vi "Flow Module (Main).vi"(7 "Name of Parent Panel":string="Main.vi", 9 "New Center Coords":T2={"Horizontal"=470, "Vertical"=200}, 10 "Config":variant, 11 "Main UI Message Queue":refnum<queue>) -> ()   [LabVIEW 2018, in "Flow Module.lvlib"]
doc: "This Continuous Measurement sample project is based on the Queued Message Handler template.\n\nThe Event Handling Loop generates messages based on user interface actions.\n\nThe Message Handling Loop processes messages generated by the Event Handling Loop, or by other messages. There are also Acquisition and Logging message handling loop subVIs, and a chart updating loop."
uses:
  Flow Module.lvlib
  support/Message Queue/Message Cluster.ctl
  <vilib>/Utility/miscctls.llb/LVPoint32TypeDef.ctl
  controls/UI State.ctl
  Feed Module/Controls/Flow Module State Cluster.ctl
  Feed Module/Controls/Flow Module Config Cluster.ctl
  Feed Module/Controls/Flow Module Settings Cluster.ctl
  Bronkhorst M13 Flow Meter/Settings Cluster.ctl
  Bronkhorst M14 Flow Meter/Settings Cluster.ctl
  Feed Module/Controls/Flow Module Display.ctl
  support/Message Queue/Enqueue Message (Single).vi
  support/User Event - Stop/User Event - Stop.lvlib
  support/Message Queue/Message Queue.lvlib
  support/Support Library.lvlib
  Measure Instrument/Flow Module Engine.lvlib
  support/Command Log VIs/Command Logging.lvlib
  Bronkhorst M14 Flow Meter/Bronkhorst M14 Flow Meter.lvlib
  Bronkhorst M13 Flow Meter/Bronkhorst M13 Flow Meter.lvlib
  Report Generation/Report Generation.lvlib
panel:
  in  "Settings Button":bool
  out "User Name":string
  out "Display Cluster":T1 {"Total g" format="%4.2f"; "C" format="%5.2f"; "kg/m^3" format="%6.1f"; "g/min" format="%4.2f"}
  out "Original Width":u32
  out "Original Height":u32
  out "H/W":dbl
  out "ScanCode":i16
  out "Log File path":path
  out "Status":string
  in  "Exit":bool
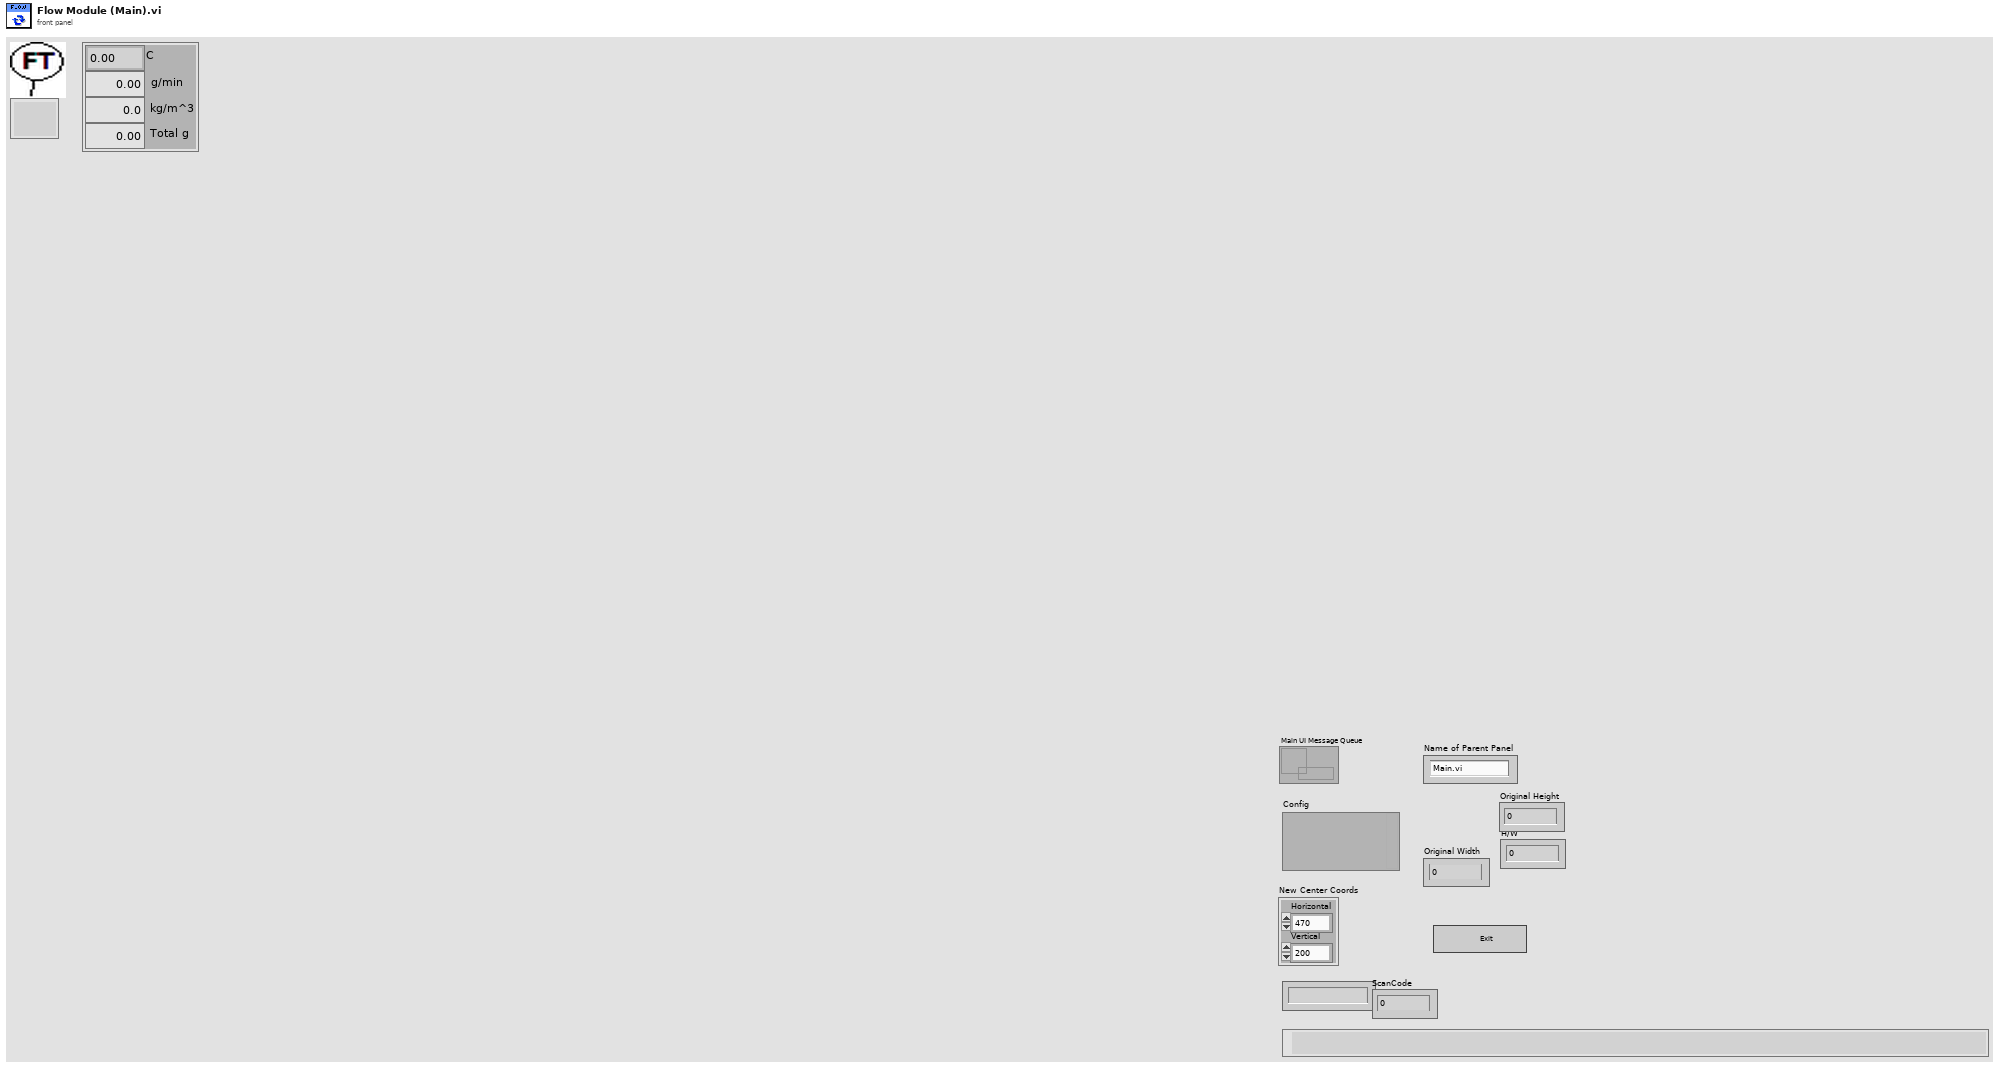
[diagram p1: front panel]
types:
  T1 = cluster{"C":dbl, "g/min":dbl, "kg/m^3":dbl, "Total g":dbl}
  T2 = typedef "LVPoint32TypeDef.ctl" = cluster{"Horizontal":i32, "Vertical":i32}
  T3 = enum32{"Invalid", "Default", "Floating", "Floating/Auto-Hide", "Modal"}
  T4 = typedef "Flow Module.lvlib/Flow Module Config Cluster.ctl" = cluster{"GUID":string, "Drop Coords":T2, "Process Name":string, "User name":string, "Queue Name":string, "Settings":T5, "Load Count":i32}
  T5 = typedef "Flow Module.lvlib/Flow Module Settings Cluster.ctl" = cluster{"Cycle Period":dbl, "Flow Meter Type":string, "Bronkhorst M13 Settings":T6, "Bronkhorst M14 Settings":T7, "Reset Totalizer":bool}
  T6 = typedef "Bronkhorst M13 Flow Meter.lvlib/Settings Cluster.ctl" = cluster{"VISA resource name":refnum<visa-resource-name>, "Simulated?":bool, "Smoothing Steps":i32}
  T7 = typedef "Bronkhorst M14 Flow Meter.lvlib/Settings Cluster.ctl" = cluster{"VISA resource name":refnum<visa-resource-name>, "Simulated?":bool, "Smoothing Steps":i32}
  T8 = typedef "UI State.ctl" = enum16{"Idle", "Acquiring and Logging", "Waiting for Exit", "Waiting for Exit (Acq Stopped)", "Waiting for Exit (Log Stopped)", "Waiting for Stop", "Waiting for Stop (Acq Stopped)", "Waiting for Stop (Log Stopped)"}
  T9 = typedef "Flow Module.lvlib/Flow Module State Cluster.ctl" = cluster{"Flow Module Config":T4}
  T10 = typedef "LVPointTypeDef.ctl" = cluster{"Horizontal":i16, "Vertical":i16}
  T11 = typedef "Flow Module.lvlib/Flow Message Queues.ctl" = cluster{"Flow UI":refnum<queue>, "Flow Engine":refnum<queue>, "Flow Display":refnum<queue>}
  T12 = typedef "Flow Module.lvlib/Flow Module Display.ctl" = cluster{"Flow Value":dbl, "Cycle Period":dbl, "Density":dbl, "Temp":dbl, "Totalized":dbl}
  T13 = typedef "LVRectTypeDef.ctl" = cluster{"Left":i16, "Top":i16, "Right":i16, "Bottom":i16}
  T14 = cluster{"Shift":bool, "Ctrl":bool, "Alt":bool, "Cmd":bool, "Opt":bool}
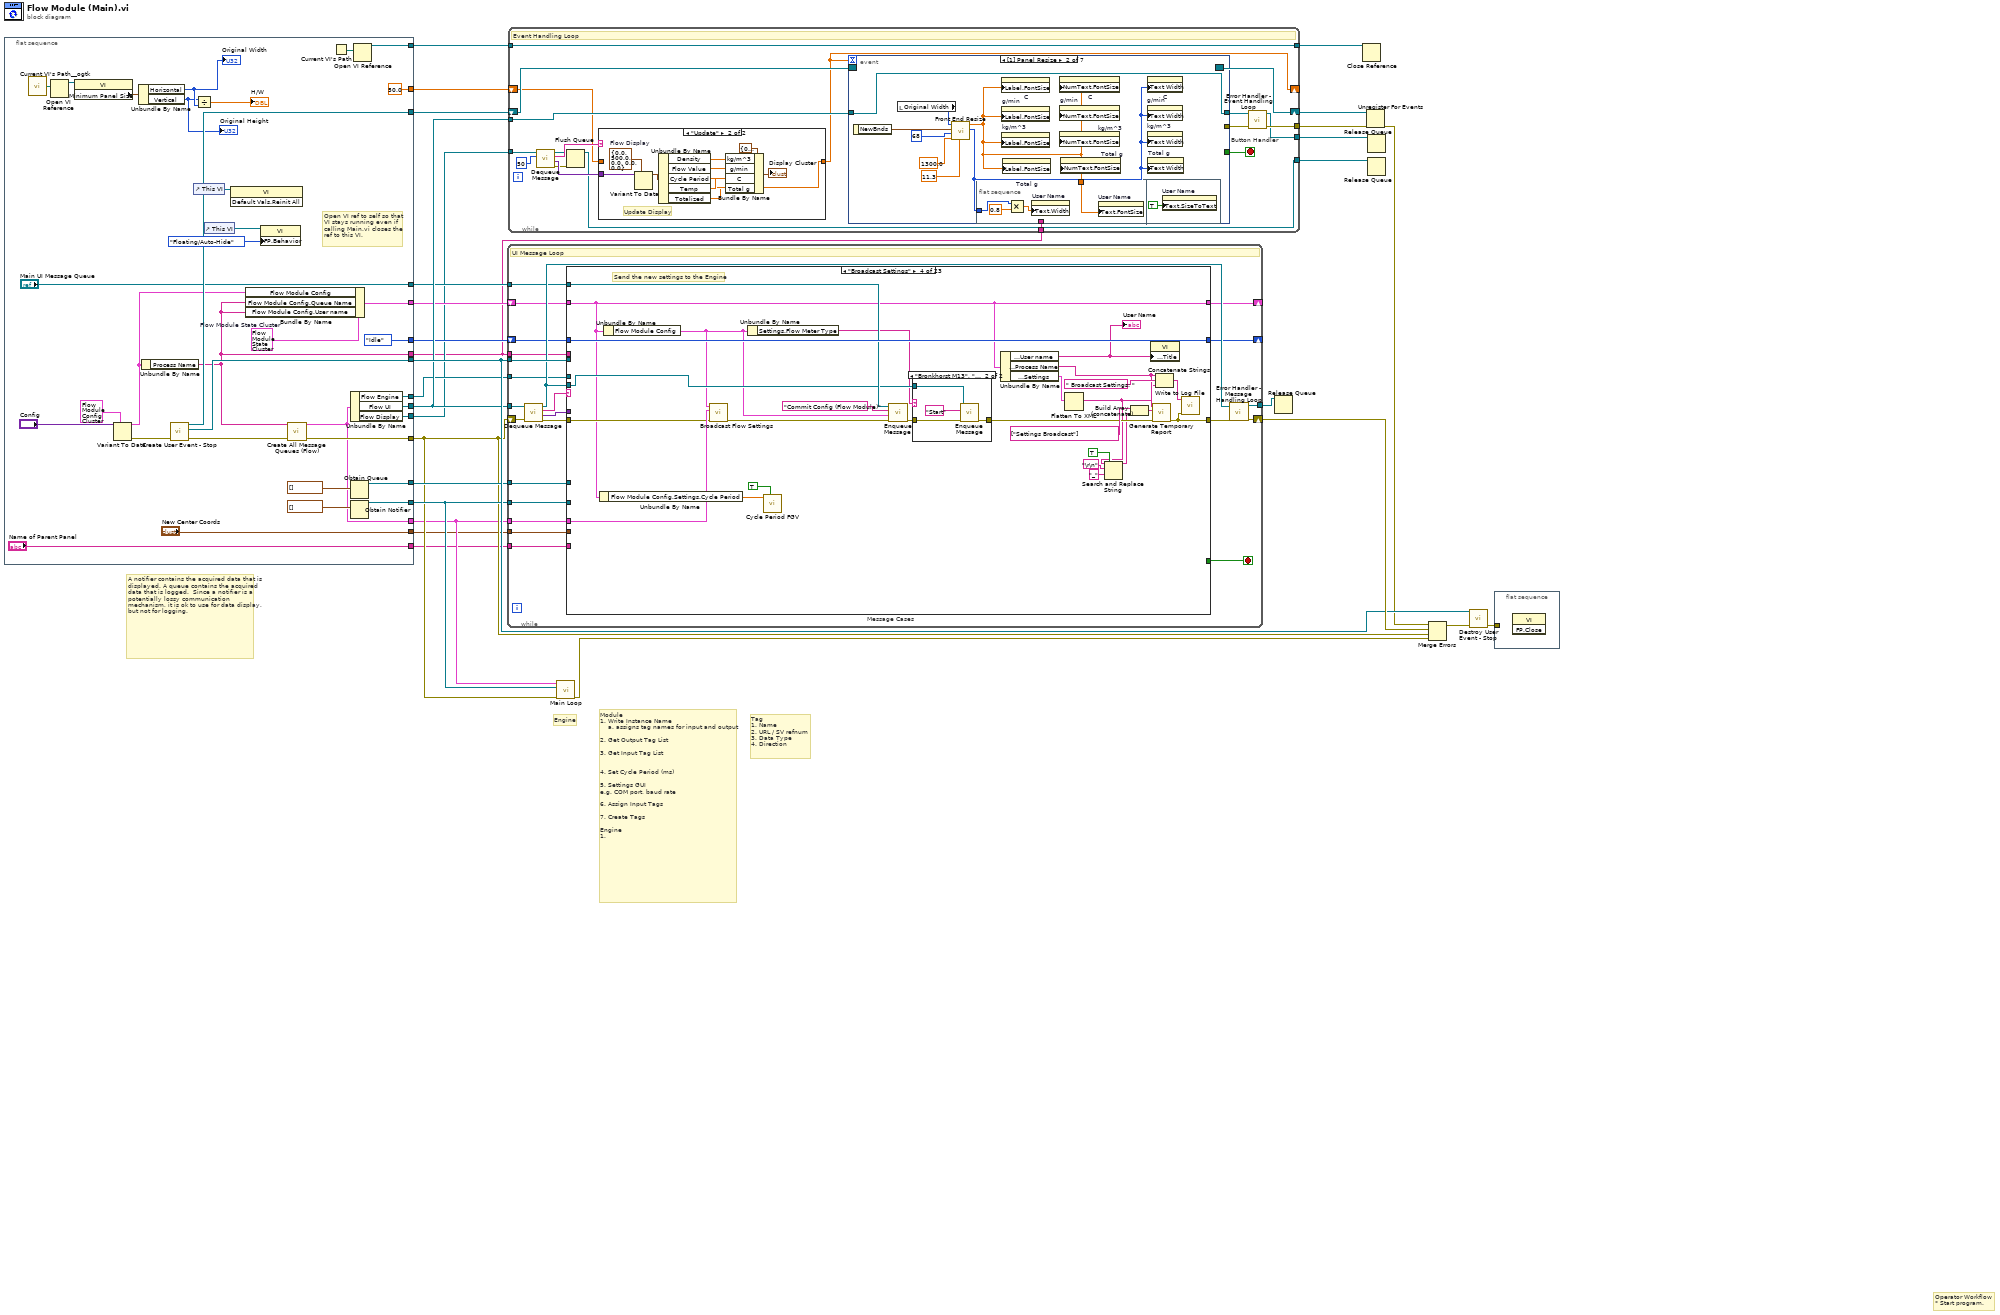
[diagram p0: block diagram]
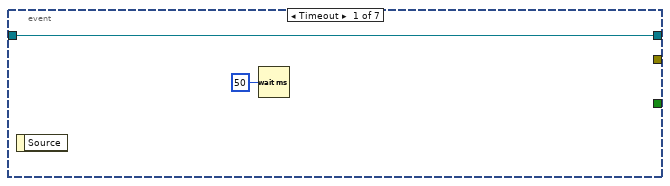
[diagram p3: hidden frame]
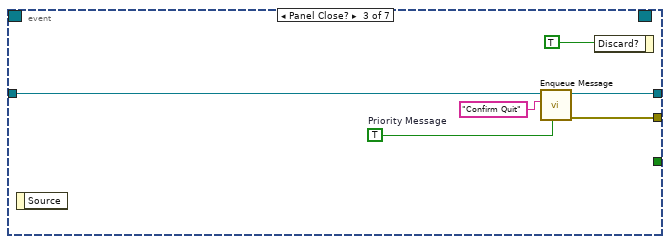
[diagram p4: hidden frame]
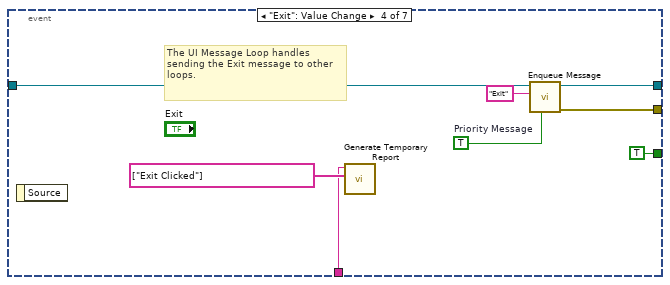
[diagram p5: hidden frame]
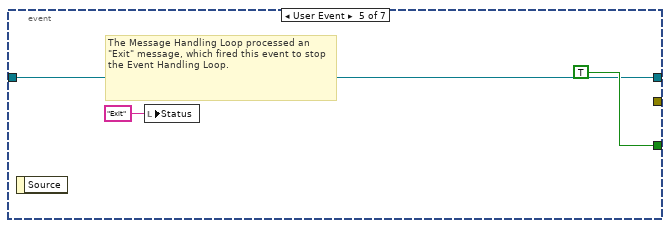
[diagram p6: hidden frame]
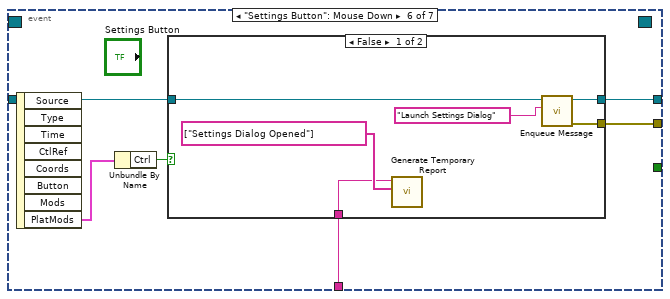
[diagram p7: hidden frame]
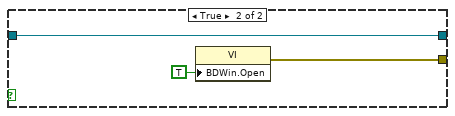
[diagram p8: hidden frame]
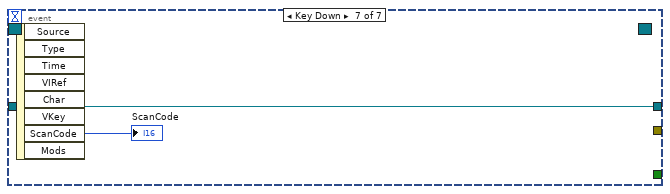
[diagram p9: hidden frame]
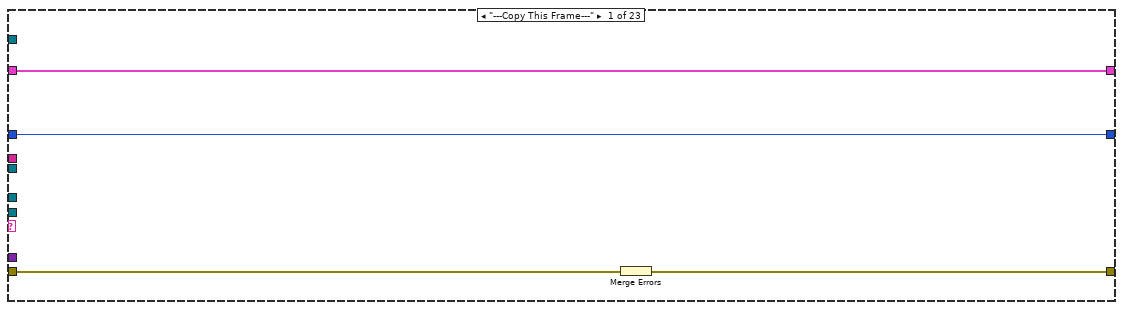
[diagram p10: hidden frame]
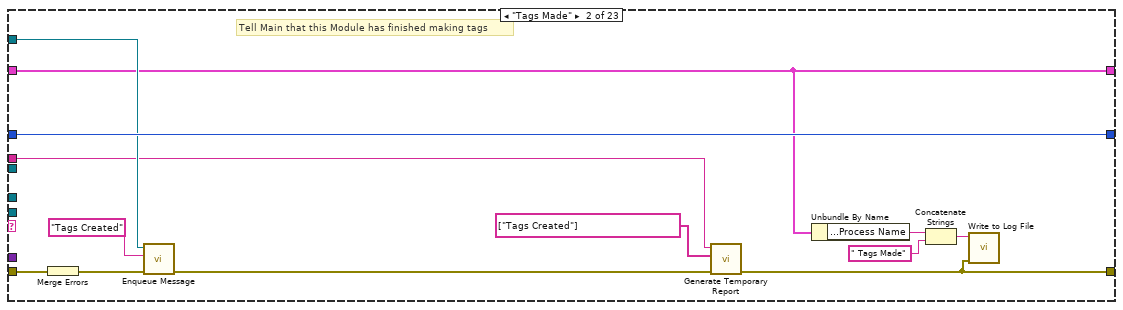
[diagram p11: hidden frame]
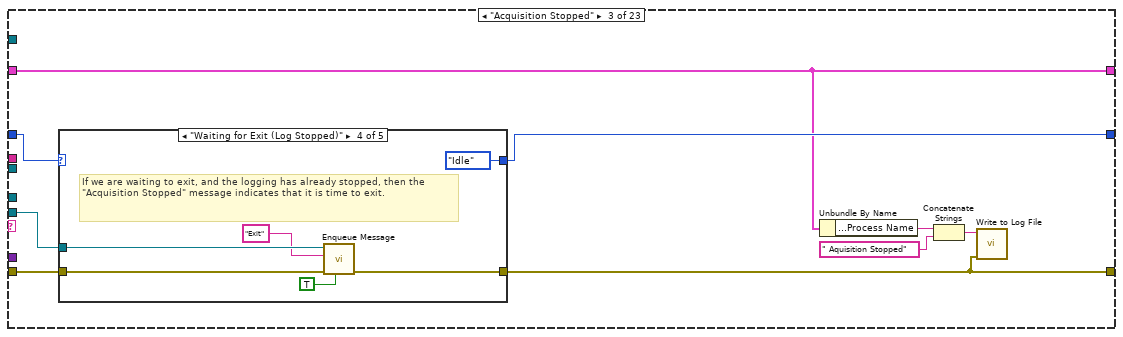
[diagram p12: hidden frame]
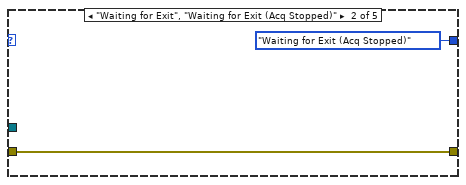
[diagram p14: hidden frame]
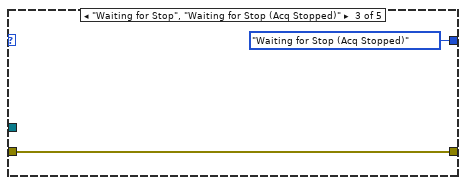
[diagram p15: hidden frame]
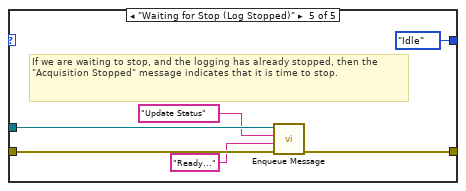
[diagram p16: hidden frame]
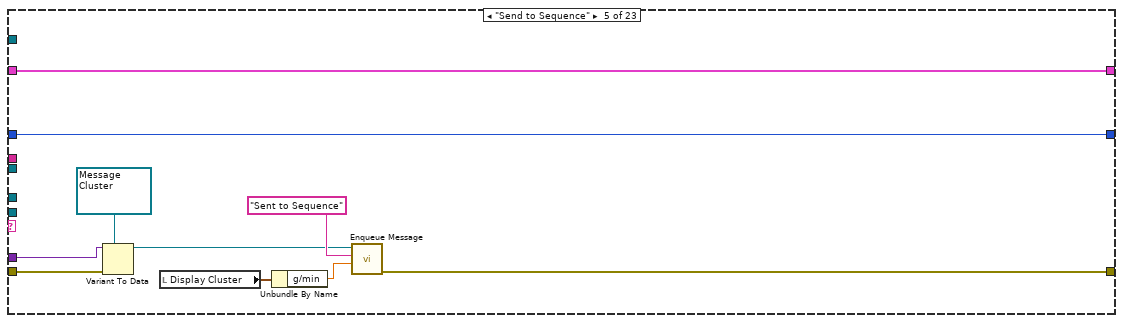
[diagram p18: hidden frame]
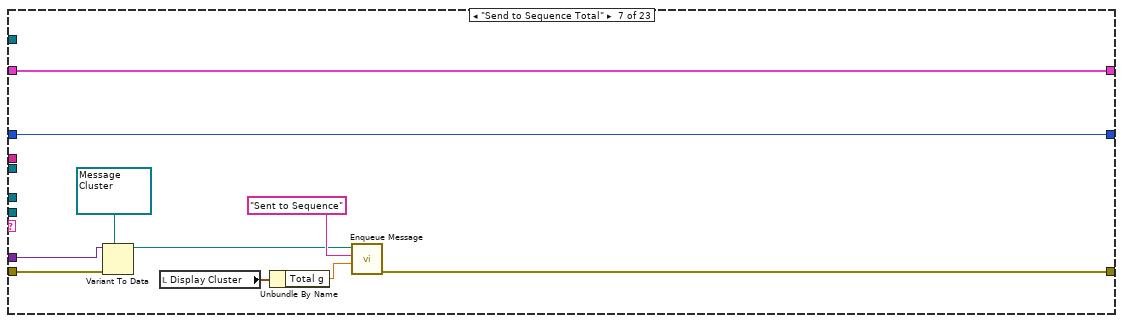
[diagram p20: hidden frame]
diagram:
  # "Engine"
  # "Operator Workflow\n* Start program."
  # "Module \n1. Write Instance Name\n    a. assigns tag names for input and output\n\n2. Get Output Tag List\n\n3. Get Input Tag List\n\n\n4. Set Cycle Period (ms)\n\n5. Settings GUI\ne.g. COM port, baud rate\n\n6. Assign Input Tags\n\n7. Create Tags\n\nEngine\n1."
  # "Tag\n1. Name\n2. URL / SV refnum\n3. Data Type\n4. Direction"
  # "A notifier contains the acquired data that is displayed. A queue contains the acquired data that is logged.  Since a notifier is a potentially lossy communication mechanism, it is ok to use for data display, but not for logging."
  n1 = flat-sequence {
    tunnel: [w63] -> w25
    tunnel: [w62] -> w24
    tunnel: [w61] -> w21
    tunnel: [UI_State."Idle" ("UI State")] -> w20
    tunnel: [w57] -> w19
    tunnel: [w56] -> w18
    tunnel: [w55] -> w16
    tunnel: [w54] -> w14
    tunnel: [w52] -> w13
    tunnel: ["Main UI Message Queue"] -> w12
    tunnel: [w48] -> w11
    tunnel: [w43] -> w10
    tunnel: [w42] -> w9
    tunnel: ["New Center Coords"] -> w8
    tunnel: ["Name of Parent Panel"] -> w7
    tunnel: [50.0 ("Cycle Period")] -> w5
    tunnel: [w35] -> w1
    frame #0 {
      w39 = T9 {"Flow Module Config"={"GUID"="PID1-Mettler Toledo Scale 1", "Drop Coords"={"Horizontal"=0, "Vertical"=0}, "Process Name"="PID1-Setpoint", "User name"="", "Queue Name"="", "Settings"={"Cycle Period"=500.0, "Flow Meter Type"="", "Bronkhorst M13 Settings"={"VISA resource name"="", "Simulated?"=FALSE, "Smoothing Steps"=1}, "Bronkhorst M14 Settings"={"VISA resource name"="", "Simulated?"=FALSE, "Smoothing Steps"=1}, "Reset Totalizer"=FALSE}, "Load Count"=0}}  # Flow Module State Cluster
      # "Open VI ref to self so that\nVI stays running even if\ncalling Main.vi closes the\nref to this VI."
      n2 = call <userlib>:"Current VI's Path__ogtk.vi"() -> ("Current VI's Path (+ Relative)"=w33:path)  [unwired: 1 in]
      n3 = Open VI Reference(vi path=w33) -> (vi reference=w32:refnum<vi>)  [unwired: 5 in, 1 out]
      n4 = property class="VI"(reference=w32) -> ("Minimum Panel Size"=w31:T10)  [unwired: 1 in, 2 out]
      n5 = Variant To Data(type=T4 {"GUID"="", "Drop Coords"={"Horizontal"=0, "Vertical"=0}, "Process Name"="", "User name"="", "Queue Name"="", "Settings"={"Cycle Period"=500.0, "Flow Meter Type"="", "Bronkhorst M13 Settings"={"VISA resource name"="", "Simulated?"=FALSE, "Smoothing Steps"=1}, "Bronkhorst M14 Settings"={"VISA resource name"="", "Simulated?"=FALSE, "Smoothing Steps"=1}, "Reset Totalizer"=FALSE}, "Load Count"=0} ("Feed Module Config"), Variant="Config") -> (data=w47:T4, error out=w51:errorcluster)  [unwired: 1 in]
      n6 = Unbundle By Name(w31) -> ("Horizontal"=w30:i16, "Vertical"=w29:i16)
      "Original Width" <- w30
      "Original Height" <- w29
      n7 = Unbundle By Name(w47) -> ("Process Name"=w35:string)
      n8 = call "Create User Event - Stop.vi"("error in (no error)"=w51) -> ("error out"=w44:errorcluster, "User Event - Stop"=w62:refnum<user-event>, "Stop Event Registration Refnum"=w63:refnum<event-registration>)  [unwired: 8 in]
      n9 = control-ref of="This VI"() -> (w46:refnum<vi>)
      n10 = Divide(x=w29, y=w30) -> (x/y=→"H/W":dbl)
      n11 = control-ref of="This VI"() -> (w37:refnum<vi>)
      n12 = invoke class="VI" method="Default Vals.Reinit All"(reference=w46) -> ()  [unwired: 2 in, 3 out]
      n13 = Bundle By Name(cluster=w39, "Flow Module Config"=w47, "Flow Module Config.Queue Name"=w35, "Flow Module Config.User name"=w35) -> (w52:T9)
      n14 = property class="VI"(reference=w37, "FP.Behavior"=T3."Floating/Auto-Hide" ("Front Panel Window:Behavior")) -> ()  [unwired: 1 in, 2 out]
      n15 = call "Create All Message Queues (Flow).vi"("error in (no error)"=w44, "Process Name"=w35) -> ("error out"=w43:errorcluster, "Message Queues"=w42:T11)  [unwired: 8 in]
      n16 = Current VI's Path() -> (path=w53:path)
      n17 = Unbundle By Name(w42) -> ("Flow Engine"=w57:refnum<queue>, "Flow UI"=w61:refnum<queue>, "Flow Display"=w48:refnum<queue>)
      n18 = Obtain Queue(element data type=waveform(dbl)[] []) -> (queue out=w56:refnum<queue>)  [unwired: 4 in, 2 out]
      n19 = Obtain Notifier(notification data type=waveform(dbl)[] []) -> (notifier out=w55:refnum<notifier>)  [unwired: 3 in, 2 out]
      n20 = Open VI Reference(vi path=w53) -> (vi reference=w54:refnum<vi>)  [unwired: 5 in, 1 out]
    }
  }
  n21 = while {
    tunnel: w21 -> [w81]
    tunnel: w24 -> [w85]
    shift-right: [w77] -> w28
    shift-left: w10 -> [w84]
    shift-right: [w68] -> _
    shift-left: w13 -> [w70]
    tunnel: w16 -> [w80]
    tunnel: w18 -> [w79]
    shift-right: [w74] -> _
    shift-left: w20 -> [w75]
    tunnel: w19 -> [w73]
    tunnel: w9 -> [w72]
    tunnel: w12 -> [w69]
    tunnel: w1 -> [w67]
    tunnel: w8 -> [w66]
    tunnel: w7 -> [w65]
    tunnel: [w64] -> w2
    stop <- w86 stop-if-true
    # "UI Message Loop"
    n22 = call "Dequeue Message.vi"("error in (no error)"=w84, "Message Queue"=w81) -> ("error out"=w71:errorcluster, "Message Data"=w82:variant, "Message"=w83:string, "dup Message Queue"=w76:refnum<queue>)  [unwired: 6 in]
    n23 = case "Message Cases" shown="\"Broadcast Settings\"" w83 {
      selector: w83 -> [_ _ _ _ _ _ _ _ _ _ _ _ _ _ _ _ _ _ _ _ _ _ w440]
      tunnel: w76 -> [_ _ w109 w149 _ _ _ w193 _ w236 w250 w274 _ w315 w331 w352 w380 _ _ _ w429 _ _]
      tunnel: w71 -> [w90 w103 w110 w153 w166 w175 w179 w192 w218 w231 w254 w273 w299 w311 w329 w353 w379 w386 w392 w410 w424 w438 _]
      tunnel: [w89 w91 w105 w134 w170 w175 w183 w187 w219 w223 w241 w255 w299 w300 w324 w348 w374 w386 w387 w403 w413 w439 w441] -> w78
      tunnel: [_ _ _ _ _ _ _ _ _ _ _ TRUE _ _ _ _ _ _ _ _ _ _ _] -> w86
      tunnel: w82 -> [_ _ _ _ w167 _ w180 _ w221 _ w253 w263 _ _ _ _ _ _ _ _ _ w437 _]
      tunnel: w85 -> [_ _ _ _ _ _ _ _ _ _ _ w284 _ _ _ _ _ _ _ _ _ _ _]
      tunnel: w70 -> [w87 w95 w104 w143 w171 w174 w184 w186 w216 w227 w240 w259 w296 w304 w323 w347 w376 w384 w393 w402 w417 w432 w446]
      tunnel: w80 -> [_ _ _ _ _ _ _ _ _ _ _ w282 _ _ _ _ _ _ _ _ _ _ _]
      tunnel: w79 -> [_ _ _ _ _ _ _ _ _ _ _ w278 _ _ _ _ _ _ _ _ _ _ _]
      tunnel: w75 -> [w88 w102 w112 w157 w172 w173 w185 w194 w217 w232 w245 w271 _ _ w333 w355 _ w385 _ _ w425 w433 w450]
      tunnel: [w88 w102 w111 w157 w172 w173 w185 w191 w217 w233 w245 w270 UI_State."Idle" ("UI State") UI_State."Idle" ("UI State") w333 w354 UI_State."Acquiring and Logging" ("UI State") w385 UI_State."Acquiring and Logging" ("UI State") UI_State."Acquiring and Logging" ("UI State") w426 w433 w450] -> w74
      tunnel: w73 -> [_ _ _ _ _ _ _ _ _ _ _ w277 _ _ _ _ _ _ w395 w408 w423 _ _]
      tunnel: w72 -> [_ _ _ w156 _ _ _ _ _ _ _ _ _ _ _ _ _ _ _ _ _ _ _]
      tunnel: w69 -> [_ w99 _ w150 _ _ _ _ _ _ _ w262 _ _ w332 _ _ _ _ _ _ _ _]
      tunnel: [w87 w95 w104 w143 w171 w174 w184 w186 w216 w227 w240 w259 w296 w304 w322 w347 w376 w384 w393 w402 w417 w432 w446] -> w68
      tunnel: w67 -> [_ w93 _ _ _ _ _ _ _ _ _ _ _ w309 _ _ _ _ _ w407 _ _ _]
      tunnel: w66 -> [_ _ _ _ _ _ _ _ _ _ _ _ _ w308 _ _ _ _ _ _ _ _ _]
      tunnel: w65 -> [_ _ _ _ _ _ _ _ _ _ _ _ _ w307 _ _ _ _ _ _ _ _ _]
      frame "---Copy This Frame---" {
        # "Duplicate this frame when creating new messages.  Change this comment in the duplicated frame to describe this message."
        n24 = Merge Errors(w90) -> (w89:errorcluster)
      }
      frame "Tags Made" {
        # "Tell Main that this Module has finished making tags"
        # "Duplicate this frame when creating new messages.  Change this comment in the duplicated frame to describe this message."
        n25 = Merge Errors(w103) -> (w100:errorcluster)
        n26 = call-poly "Enqueue Message.vi"("error in (no error)"=w100, "Message"="Tags Created", "Message Queue"=w99) -> ("error out"=w92:errorcluster)  [unwired: 7 in, 1 out]
        n27 = call "Generate Temporary Report.vi"("error in (no error)"=w92, "Line of Events"=string[] ["Tags Created"], "Module Name"=w93) -> ("error out"=w91:errorcluster)  [unwired: 8 in]
        n28 = Unbundle By Name(w95) -> ("Flow Module Config.Process Name"=w98:string)
        n29 = Concatenate Strings(w98, " Tags Made" ("text")) -> (w96:string)
        n30 = call "Write to Log File.vi"("error in"=w91, "text"=w96) -> ()  [unwired: 9 in, 1 out]
      }
      frame "Acquisition Stopped" {
        # "Logic for determining what action to take when the acquisition has stopped."
        n31 = case shown="\"Waiting for Exit (Log Stopped)\"" w112 {
          selector: w112 -> [w114 _ _ _ _]
          tunnel: [w114 UI_State."Waiting for Exit (Acq Stopped)" ("UI State") UI_State."Waiting for Stop (Acq Stopped)" ("UI State") UI_State."Idle" ("UI State") UI_State."Idle" ("UI State")] -> w111
          tunnel: w110 -> [w113 w115 w117 w123 w129]
          tunnel: [w113 w115 w117 w122 w128] -> w105
          tunnel: w109 -> [_ _ _ w121 w127]
          frame Default {
          }
          frame "Waiting for Exit", "Waiting for Exit (Acq Stopped)" {
          }
          frame "Waiting for Stop", "Waiting for Stop (Acq Stopped)" {
          }
          frame "Waiting for Exit (Log Stopped)" {
            # "If we are waiting to exit, and the logging has already stopped, then the \"Acquisition Stopped\" message indicates that it is time to exit."
            n32 = call-poly "Enqueue Message.vi"("Priority Message? (F)"=TRUE, "error in (no error)"=w123, "Message"="Exit", "Message Queue"=w121) -> ("error out"=w122:errorcluster)  [unwired: 6 in, 1 out]
          }
          frame "Waiting for Stop (Log Stopped)" {
            # "If we are waiting to stop, and the logging has already stopped, then the \"Acquisition Stopped\" message indicates that it is time to stop."
            n33 = call-poly "Enqueue Message.vi"("error in (no error)"=w129, "Message Data"="Ready..." ("Message"), "Message"="Update Status", "Message Queue"=w127) -> ("error out"=w128:errorcluster)  [unwired: 6 in, 1 out]
          }
        }
        n34 = Unbundle By Name(w104) -> ("Flow Module Config.Process Name"=w108:string)
        n35 = Concatenate Strings(w108, " Aquisition Stopped" ("text")) -> (w106:string)
        n36 = call "Write to Log File.vi"("error in"=w105, "text"=w106) -> ()  [unwired: 9 in, 1 out]
      }
      frame "Broadcast Settings" {
        # "Send the new settings to the Engine"
        # "Send the 'Update Settings' message to the Logging and Acquisition message loops."
        n37 = Unbundle By Name(w143) -> ("Flow Module Config.Settings.Cycle Period"=w154:dbl)
        n38 = Unbundle By Name(w143) -> ("Flow Module Config"=w146:T4)
        n39 = call "Broadcast Flow Settings.vi"("error in (no error)"=w153, "Message Queues"=w156, "Flow Module Config"=w146) -> ("error out"=w151:errorcluster)  [unwired: 8 in]
        n40 = Unbundle By Name(w146) -> ("Settings.Flow Meter Type"=w147:string)
        n41 = call "Cycle Period FGV.vi"("Write"=TRUE, "Cycle Period In (ms)"=w154) -> ()  [unwired: 8 in, 2 out]
        n42 = call-poly "Enqueue Message.vi"("error in (no error)"=w151, "Message Data"=w146, "Message"="Commit Config (Flow Module)", "Message Queue"=w150) -> ("error out"=w148:errorcluster)  [unwired: 6 in, 1 out]
        n43 = case shown="\"Bronkhorst M13\", \"Bronkhorst M14\"" w147 {
          tunnel: w149 -> [_ w161]
          tunnel: w148 -> [w158 w160]
          tunnel: [w158 w159] -> w135
          frame "False", Default {
          }
          frame "Bronkhorst M13", "Bronkhorst M14" {
            n44 = call-poly "Enqueue Message.vi"("error in (no error)"=w160, "Message"="Start", "Message Queue"=w161) -> ("error out"=w159:errorcluster)  [unwired: 7 in, 1 out]
          }
        }
        n45 = Unbundle By Name(w143) -> ("Flow Module Config.User name"=w131:string, "Flow Module Config.Process Name"=w136:string, "Flow Module Config.Settings"=w142:T5)
        "User Name" <- w131
        n46 = Flatten To XML(anything=w142) -> (xml string=w133:string)
        n47 = Search and Replace String(replace all?=TRUE ("replace all? (F)"), input string=w133, search string="\r\n", replace string="_" ("replace string (\"\")")) -> (result string=w132:string)  [unwired: 4 in, 3 out]
        n48 = Build Array (concatenate)(string[] ["Settings Broadcast"] ("Line of Events"), w132) -> (w137:string[])
        n49 = property class="VI"("Front Panel.Title"=w131) -> ()  [unwired: 2 in, 2 out]
        n50 = call "Generate Temporary Report.vi"("error in (no error)"=w135, "Line of Events"=w137, "Module Name"=w136) -> ("error out"=w134:errorcluster)  [unwired: 8 in]
        n51 = Concatenate Strings(w136, " Broadcast Settings: " ("text"), w133) -> (w144:string)
        n52 = call "Write to Log File.vi"("error in"=w134, "text"=w144) -> ()  [unwired: 9 in, 1 out]
      }
      frame "Send to Sequence" {
        n53 = Variant To Data(error in=w166, type=refnum<queue> refnum ("Message Queue"), Variant=w167) -> (data=w165:refnum<queue>)  [unwired: 1 out]
        n54 = local read "Display Cluster"() -> (w164:T1)
        n55 = Unbundle By Name(w164) -> ("g/min"=w163:dbl)
        n56 = call-poly "Enqueue Message.vi"("Message Data"=w163, "Message"="Sent to Sequence", "Message Queue"=w165) -> ("error out"=w170:errorcluster)  [unwired: 7 in, 1 out]
      }
      frame "Sequence Update" {
      }
      frame "Send to Sequence Total" {
        n57 = Variant To Data(error in=w179, type=refnum<queue> refnum ("Message Queue"), Variant=w180) -> (data=w178:refnum<queue>)  [unwired: 1 out]
        n58 = local read "Display Cluster"() -> (w177:T1)
        n59 = Unbundle By Name(w177) -> ("Total g"=w176:dbl)
        n60 = call-poly "Enqueue Message.vi"("Message Data"=w176, "Message"="Sent to Sequence", "Message Queue"=w178) -> ("error out"=w183:errorcluster)  [unwired: 7 in, 1 out]
      }
      frame "Confirm Quit" {
        # "Confirm Quit - Message that can confirm whether or not the user wants to exit the application."
        n61 = case shown="Default" w194 {
          tunnel: w193 -> [w199 w205]
          tunnel: w192 -> [w198 w203]
          tunnel: [w195 w202] -> w187
          tunnel: [UI_State."Idle" ("UI State") w201] -> w191
          frame Default {
            # "If 'Confirm Quit' comes in while the system is idle, there is no need for a confirmation message."
            n62 = call-poly "Enqueue Message.vi"("Priority Message? (F)"=TRUE, "error in (no error)"=w198, "Message"="Exit", "Message Queue"=w199) -> ("error out"=w195:errorcluster)  [unwired: 6 in, 1 out]
          }
          frame "Acquiring and Logging" {
            n63 = Two Button Dialog(message="Are you sure you want to quit while the acquisition is running?" ("Confirm Quit Message"), 1:"No" ("No"), 2:"Yes" ("Yes")) -> (T button?=w204:bool)
            n64 = case shown="True" w204 {
              tunnel: w205 -> [_ w215]
              tunnel: w203 -> [w209 w214]
              tunnel: [w209 w213] -> w202
              tunnel: [UI_State."Acquiring and Logging" ("UI State") UI_State."Waiting for Exit" ("UI State")] -> w201
              frame False {
                # "User did not want to quit."
              }
              frame True {
                n65 = call-poly "Enqueue Message.vi"("error in (no error)"=w214, "Message"="Exit", "Message Queue"=w215) -> ("error out"=w213:errorcluster)  [unwired: 7 in, 1 out]
              }
            }
          }
        }
        n66 = Unbundle By Name(w186) -> ("Flow Module Config.Process Name"=w190:string)
        n67 = Concatenate Strings(w190, " Quit" ("text")) -> (w188:string)
        n68 = call "Write to Log File.vi"("error in"=w187, "text"=w188) -> ()  [unwired: 9 in, 1 out]
      }
      frame "Display Log File Path" {
        n69 = Variant To Data(error in=w218, type=path "", Variant=w221) -> (data=→"Log File path":path, error out=w219:errorcluster)
      }
      frame "E-Stop" {
        # "Doesn't really do anything because this is just a read module"
        # "Message Acquisition and Logging loops to stop"
        # "Stop the pumps."
        n70 = call-poly "Enqueue Message.vi"("error in (no error)"=w231, "Message Data"="Ready..." ("Ready..."), "Message"="Update Status", "Message Queue"=w236) -> ("error out"=w230:errorcluster)  [unwired: 6 in, 1 out]
        n71 = case shown="\"Waiting for Exit\"" w232 {
          selector: w232 -> [_ w238]
          tunnel: [UI_State."Waiting for Stop" ("UI State") w238] -> w233
          frame Default {
          }
          frame "Waiting for Exit" {
          }
        }
        n72 = Merge Errors(w230) -> (w224:errorcluster)
        n73 = Unbundle By Name(w227) -> ("Flow Module Config.Process Name"=w225:string)
        n74 = call "Generate Temporary Report.vi"("error in (no error)"=w224, "Line of Events"=string[] ["E-STOP"], "Module Name"=w225) -> ("error out"=w223:errorcluster)  [unwired: 8 in]
        n75 = Concatenate Strings(w225, " E-STOP" ("text")) -> (w228:string)
        n76 = call "Write to Log File.vi"("error in"=w223, "text"=w228) -> ()  [unwired: 9 in, 1 out]
      }
      frame "Error" {
        # "Exit on error"
        # "Error - Check the error message data and respond accordingly. This message is sent by the \"Error Handler\" VIs at the end of each loop in this application."
        n77 = Variant To Data(error in=w254, type=errorcluster {"status"=FALSE, "code"=0, "source"=""} ("error out"), Variant=w253) -> (data=w251:errorcluster, error out=w247:errorcluster)
        n78 = call <vilib>:"General Error Handler.vi"("error in (no error)"=w251) -> ("message"=w239:string)  [unwired: 10 in, 4 out]
        n79 = call-poly "Enqueue Message.vi"("Priority Message? (F)"=TRUE, "Message"="Exit", "Message Queue"=w250) -> ("error out"=w246:errorcluster)  [unwired: 7 in, 1 out]
        n80 = Merge Errors(w246, w247) -> (w241:errorcluster)
        n81 = Unbundle By Name(w240) -> ("Flow Module Config.Process Name"=w244:string)
        n82 = Concatenate Strings(w244, " Error: " ("text"), w239) -> (w242:string)
        n83 = call "Write to Log File.vi"("error in"=w241, "text"=w242) -> ()  [unwired: 9 in, 1 out]
      }
      frame "Exit" {
        w266 = TRUE  # Delete Module?
        # "Don't check the error outs. The acquisition and logging queues may have already been released."
        # "Close references owned by the Main VI."
        # "Stop the VI"
        # "Exit - Fire the User Event to stop the Event Handling Loop.  Also send Exit messages to the Acquisition and Logging loops."
        n84 = Build Array(w277) -> (w276:refnum<queue>[])
        n85 = Variant To Data(type=w266, Variant=w263) -> (data=w265:bool, error out=w267:errorcluster)  [unwired: 1 in]
        n86 = Select(t=w266, s=w267, f=w265) -> (s? t:f=w264:bool)
        n87 = for {
          tunnel: w276 -> [w293] mode=indexing
          # "Stop Logging and Exit"
          n88 = call-poly "Enqueue Message.vi"("Message"="Stop", "Message Queue"=w293) -> ("dup Message Queue"=w294:refnum<queue>)  [unwired: 8 in, 1 out]
          n89 = call-poly "Enqueue Message.vi"("Message"="Exit", "Message Queue"=w294) -> ()  [unwired: 8 in, 2 out]
        }
        n90 = case "Don't enqueue Delete Module if opening campaign because it\nwill already have been deleted and new config loaded and we create\na race condition." shown="True" w264 {
          tunnel: w262 -> [_ w288]
          tunnel: w259 -> [_ w287]
          frame False {
          }
          frame True {
            n91 = Unbundle By Name(w287) -> ("Flow Module Config.GUID"=w286:string)
            n92 = call-poly "Enqueue Message.vi"("Message Data"=w286, "Message"="Delete Module", "Message Queue"=w288) -> ()  [unwired: 7 in, 2 out]
          }
        }
        n93 = call-poly "Enqueue Message.vi"("error in (no error)"=w273, "Message Data"="Ready..." ("Ready..."), "Message"="Update Status", "Message Queue"=w274) -> ("error out"=w272:errorcluster, "dup Message Queue"=w269:refnum<queue>)  [unwired: 6 in]
        n94 = Release Queue(queue=w269, error in (no error)=w272) -> (error out=w281:errorcluster)  [unwired: 1 in, 2 out]
        n95 = Release Notifier(notifier=w282, error in (no error)=w281) -> (error out=w280:errorcluster)  [unwired: 1 in, 2 out]
        n96 = call "Fire User Event - Stop.vi"("User Event - Stop"=w284) -> ("error out"=w283:errorcluster)  [unwired: 10 in]
        n97 = Release Queue(queue=w278, error in (no error)=w280) -> (error out=w279:errorcluster)  [unwired: 1 in, 2 out]
        n98 = case shown="Default" w271 {
          selector: w271 -> [_ w291]
          tunnel: [UI_State."Waiting for Stop" ("UI State") w291] -> w270
          frame Default {
          }
          frame "Waiting for Exit" {
          }
        }
        n99 = Merge Errors(w283, w279) -> (w256:errorcluster)
        n100 = Unbundle By Name(w259) -> ("Flow Module Config.Process Name"=w257:string)
        n101 = Concatenate Strings(w257, " Exit" ("text")) -> (w260:string)
        n102 = call "Generate Temporary Report.vi"("error in (no error)"=w256, "Line of Events"=string[] ["Exited"], "Module Name"=w257) -> ("error out"=w255:errorcluster)  [unwired: 8 in]
        n103 = call "Write to Log File.vi"("error in"=w255, "text"=w260) -> ()  [unwired: 9 in, 1 out]
      }
      frame "Init UI Refs" {
        # "Init UI Refs - Store control references for UI controls.  Also enable/disable controls appropriately."
        n104 = property class="VI"("Front Panel.Closeable"=TRUE ("Front Panel Window:Closeable")) -> ()  [unwired: 2 in, 2 out]
      }
      frame "Initialize" {
        # "Initialize - Get configuration settings, then message the UI to initialize, and broadcast the settings to the other message loops."
        n105 = property class="VI" props=["FP.State"]() -> (reference out=w310:refnum<vi>)  [unwired: 2 in, 2 out]
        n106 = call-poly "Enqueue Message.vi"("error in (no error)"=w311, "Message"="Init UI Refs", "Message Queue"=w315) -> ("error out"=w313:errorcluster, "dup Message Queue"=w314:refnum<queue>)  [unwired: 7 in]
        n107 = call "Make Child and Move.vi"("Process Name"=w309, "Name of Parent Panel"=w307, "New Center Coords"=w308, "VI in"=w310) -> ()  [unwired: 8 in]
        n108 = call-poly "Enqueue Message.vi"("error in (no error)"=w313, "Message"="Broadcast Settings", "Message Queue"=w314) -> ("error out"=w321:errorcluster, "dup Message Queue"=w320:refnum<queue>)  [unwired: 7 in]
        n109 = call-poly "Enqueue Message.vi"("error in (no error)"=w321, "Message Data"="Ready..." ("Ready..."), "Message"="Update Status", "Message Queue"=w320) -> ("error out"=w301:errorcluster)  [unwired: 6 in, 1 out]
        n110 = Unbundle By Name(w304) -> ("Flow Module Config.Process Name"=w302:string)
        n111 = call "Generate Temporary Report.vi"("error in (no error)"=w301, "Line of Events"=string[] ["Initialize"], "Module Name"=w302) -> ("error out"=w300:errorcluster)  [unwired: 8 in]
        n112 = Concatenate Strings(w302, " Initialize" ("text")) -> (w305:string)
        n113 = call "Write to Log File.vi"("error in"=w300, "text"=w305) -> ()  [unwired: 9 in, 1 out]
      }
      frame "Launch Settings Dialog" {
        # "Launch the Settings Dialog when the user clicks the 'Settings' button."
        n114 = in-place {
          in-place-border: [w339] -> w330
          in-place-border: w329 -> [w338]
          in-place-border: [w337] -> w328
          # "Keep track of the # of times the dialog has been opened"
          n115 = in-place-cluster #1(w323) -> ("Flow Module Config"=w335:T4)
          n116 = in-place {
            n117 = in-place-cluster #2(w335) -> ("Load Count"=w340:i32)
            n118 = Increment(x=w340) -> (x+1=w341:i32)
            n119 = in-place-cluster #2("Load Count"=w341) -> (w334:T4)
          }
          n120 = call "Flow Settings Dialog.vi"("error in (no error)"=w338, "Flow Module Config In"=w334) -> ("error out"=w339:errorcluster, "UI Refresh Needed?"=w337:bool, "Flow Module Config Out"=w336:T4)  [unwired: 6 in, 1 out]
          n121 = in-place-cluster #1("Flow Module Config"=w336) -> (w322:T9)
        }
        n122 = case shown="False" w328 {
          tunnel: w330 -> [w343 w346]
          tunnel: [w342 w346] -> w324
          tunnel: w332 -> [_ _]
          tunnel: w331 -> [w345 _]
          frame False {
            n123 = call-poly "Enqueue Message.vi"("error in (no error)"=w343, "Message"="Broadcast Settings", "Message Queue"=w345) -> ("error out"=w342:errorcluster)  [unwired: 7 in, 1 out]
          }
          frame True {
          }
        }
        n124 = Unbundle By Name(w322) -> ("Flow Module Config.Process Name"=w327:string)
        n125 = Concatenate Strings(w327, " Settings Dialog Launched" ("text")) -> (w325:string)
        n126 = call "Write to Log File.vi"("error in"=w324, "text"=w325) -> ()  [unwired: 9 in, 1 out]
      }
      frame "Logging Stopped" {
        # "Logic for determining what action to take when the logging has stopped."
        n127 = case shown="\"Waiting for Exit (Acq Stopped)\"" w355 {
          selector: w355 -> [w357 _ _ _ _]
          tunnel: [w357 UI_State."Waiting for Exit (Log Stopped)" ("UI State") UI_State."Waiting for Stop (Log Stopped)" ("UI State") UI_State."Idle" ("UI State") UI_State."Idle" ("UI State")] -> w354
          tunnel: w353 -> [w356 w358 w360 w366 w372]
          tunnel: [w356 w358 w360 w365 w371] -> w348
          tunnel: w352 -> [_ _ _ w364 w370]
          frame Default {
          }
          frame "Waiting for Exit", "Waiting for Exit (Log Stopped)" {
          }
          frame "Waiting for Stop", "Waiting for Stop (Log Stopped)" {
          }
          frame "Waiting for Exit (Acq Stopped)" {
            # "If we are waiting to exit, and the acquisition has already stopped, then the \"Logging Stopped\" message indicates that it is time to exit."
            n128 = call-poly "Enqueue Message.vi"("Priority Message? (F)"=TRUE, "error in (no error)"=w366, "Message"="Exit", "Message Queue"=w364) -> ("error out"=w365:errorcluster)  [unwired: 6 in, 1 out]
          }
          frame "Waiting for Stop (Acq Stopped)" {
            # "If we are waiting to stop, and the acquisition has already stopped, then the \"Logging Stopped\" message indicates that it is time to stop."
            n129 = call-poly "Enqueue Message.vi"("error in (no error)"=w372, "Message Data"="Ready..." ("Message"), "Message"="Update Status", "Message Queue"=w370) -> ("error out"=w371:errorcluster)  [unwired: 6 in, 1 out]
          }
        }
        n130 = Unbundle By Name(w347) -> ("Flow Module Config.Process Name"=w351:string)
        n131 = Concatenate Strings(w351, " Logging Stopped" ("text")) -> (w349:string)
        n132 = call "Write to Log File.vi"("error in"=w348, "text"=w349) -> ()  [unwired: 9 in, 1 out]
      }
      frame "Start" {
        # "There is only one loop but i am keeping it in for now"
        # "Message Acquisition and Logging loops to start"
        # "Start - Enable/Disable buttons appropriately for an acquisition that has started, and update status display."
        n133 = call-poly "Enqueue Message.vi"("error in (no error)"=w379, "Message"="Start Loops", "Message Queue"=w380) -> ("error out"=w381:errorcluster)  [unwired: 7 in, 1 out]
        n134 = Merge Errors(w381) -> (w374:errorcluster)
        n135 = Unbundle By Name(w376) -> ("Flow Module Config.Process Name"=w375:string)
        n136 = Concatenate Strings(w375, " Start" ("text")) -> (w377:string)
        n137 = call "Write to Log File.vi"("error in"=w374, "text"=w377) -> ()  [unwired: 9 in, 1 out]
      }
      frame "Sequence Start" {
      }
      frame "Start Loops" {
        # "I'm not sure how you could have multiple Process names in one Module"
        # "Message Acquisition and Logging loops to start"
        # "Start - Enable/Disable buttons appropriately for an acquisition that has started, and update status display."
        n138 = Unbundle By Name(w393) -> ("Flow Module Config.Process Name"=w389:string)
        n139 = Build Array(w395) -> (w394:refnum<queue>[])
        n140 = for {
          tunnel: w392 -> [w400]
          tunnel: [w399] -> w391 mode=indexing
          tunnel: w394 -> [w398] mode=indexing
          tunnel: w389 -> [w397]
          n141 = call-poly "Enqueue Message.vi"("error in (no error)"=w400, "Message Data"=w397, "Message"="Start", "Message Queue"=w398) -> ("error out"=w399:errorcluster)  [unwired: 6 in, 1 out]
        }
        n142 = Merge Errors(w392, w391) -> (w388:errorcluster)
        n143 = call "Generate Temporary Report.vi"("error in (no error)"=w388, "Line of Events"=string[] ["Started"], "Module Name"=w389) -> ("error out"=w387:errorcluster)  [unwired: 8 in]
      }
      frame "Start Log" {
        # "Message Acquisition and Logging loops to start"
        # "Start - Enable/Disable buttons appropriately for an acquisition that has started, and update status display."
        n144 = call-poly "Enqueue Message.vi"("error in (no error)"=w410, "Message Data"=w407, "Message"="Start Log", "Message Queue"=w408) -> ("error out"=w411:errorcluster)  [unwired: 6 in, 1 out]
        n145 = Merge Errors(w411) -> (w403:errorcluster)
        n146 = Unbundle By Name(w402) -> ("Flow Module Config.Process Name"=w406:string)
        n147 = Concatenate Strings(w406, " Start Log" ("text")) -> (w404:string)
        n148 = call "Write to Log File.vi"("error in"=w403, "text"=w404) -> ()  [unwired: 9 in, 1 out]
      }
      frame "Stop" {
        # "Stop - Enable/Disable buttons appropriately for an acquisition that has stopped, and update status display."
        n149 = call-poly "Enqueue Message.vi"("error in (no error)"=w424, "Message Data"="Ready..." ("Ready..."), "Message"="Update Status", "Message Queue"=w429) -> ("error out"=w422:errorcluster)  [unwired: 6 in, 1 out]
        n150 = call-poly "Enqueue Message.vi"("error in (no error)"=w422, "Message"="Stop", "Message Queue"=w423) -> ("error out"=w420:errorcluster)  [unwired: 7 in, 1 out]
        n151 = case shown="Default" w425 {
          selector: w425 -> [_ w431]
          tunnel: [UI_State."Waiting for Stop" ("UI State") w431] -> w426
          frame Default {
          }
          frame "Waiting for Exit" {
          }
        }
        n152 = Merge Errors(w420) -> (w414:errorcluster)
        n153 = Unbundle By Name(w417) -> ("Flow Module Config.Process Name"=w415:string)
        n154 = call "Generate Temporary Report.vi"("error in (no error)"=w414, "Line of Events"=string[] ["Stopped"], "Module Name"=w415) -> ("error out"=w413:errorcluster)  [unwired: 8 in]
        n155 = Concatenate Strings(w415, " Stop" ("text")) -> (w418:string)
        n156 = call "Write to Log File.vi"("error in"=w413, "text"=w418) -> ()  [unwired: 9 in, 1 out]
      }
      frame "Update Status" {
        # "Update Display - Convert the message data to a string to display in the Status indicator."
        n157 = Variant To Data(error in=w438, type="", Variant=w437) -> (data=→"Status":string, error out=w435:errorcluster)
        n158 = Merge Errors(w435) -> (w439:errorcluster)
      }
      frame Default {
        # "'Default' case only runs if there is a message that isn't defined in any of the other cases.  Output a programming error."
        n159 = Concatenate Strings("The invalid message string " ("string"), w440, " was received in Feed Module Main." ("string")) -> (w442:string)
        n160 = Bundle By Name(cluster=errorcluster {"status"=TRUE, "code"=1, "source"=""} ("error constant"), "source"=w442) -> (w441:errorcluster)
        n161 = Unbundle By Name(w446) -> ("Flow Module Config.Process Name"=w449:string)
        n162 = Concatenate Strings(w449, "Incorrect Message recieved: " ("text"), w440) -> (w447:string)
        n163 = call "Write to Log File.vi"("error in"=w441, "text"=w447) -> ()  [unwired: 9 in, 1 out]
      }
    }
    n164 = call "Error Handler - Message Handling Loop.vi"("error in (no error)"=w78, "Message Queue"=w76) -> ("dup error in"=w77:errorcluster, "dup Message Queue"=w64:refnum<queue>)  [unwired: 8 in]
  }
  n165 = while {
    tunnel: w21 -> [w463]
    tunnel: [w465] -> w27
    shift-right: [w464] -> w22
    shift-left: w25 -> [w469]
    tunnel: [w462] -> w15
    tunnel: w14 -> [w462]
    tunnel: w11 -> [w461]
    shift-right: [w458] -> _
    shift-left: w5 -> [w457]
    tunnel: [w453] -> w4
    tunnel: [w452] -> w3
    tunnel: w1 -> [w451]
    stop <- w468 stop-if-true
    # "Event Handling Loop"
    n166 = call "Dequeue Message.vi"("timeout in ms (-1)"=50, "Message Queue"=w461) -> ("error out"=w454:errorcluster, "Message Data"=w459:variant, "Message"=w460:string, "dup Message Queue"=w455:refnum<queue>)  [unwired: 6 in]
    n167 = Flush Queue(queue=w455, error in (no error)=w454) -> (queue out=w452:refnum<queue>)  [unwired: 2 out]
    n168 = case shown="\"Update\"" w460 {
      tunnel: w459 -> [_ w480]
      tunnel: [w470 w474] -> w458
      tunnel: w457 -> [w470 _]
      frame "False", Default {
      }
      frame "Update" {
        w478 = T12 {"Flow Value"=0.0, "Cycle Period"=500.0, "Density"=0.0, "Temp"=0.0, "Totalized"=0.0}  # Flow Display
        # "Update Display"
        n169 = Variant To Data(type=w478, Variant=w480) -> (data=w479:T12)  [unwired: 1 in, 1 out]
        n170 = Unbundle By Name(w479) -> ("Density"=w477:dbl, "Flow Value"=w476:dbl, "Cycle Period"=w474:dbl, "Temp"=w475:dbl, "Totalized"=w471:dbl)
        n171 = Bundle By Name(cluster=T1 {"C"=0.0, "g/min"=0.0, "kg/m^3"=0.0, "Total g"=0.0} ("Display Cluster"), "kg/m^3"=w477, "g/min"=w476, "C"=w475, "Total g"=w471) -> (→"Display Cluster":T1)
      }
    }
    n172 = event "Button Handler" shown="[1] Panel Resize" {
      selector: w469 -> [_ _ _ _ _ _ _]
      dyn-events: [_ _ _ _ _ _ _] -> w464
      timeout: w458 -> [_ _ _ _ _ _ _]
      tunnel: [_ _ _ TRUE ("Discard?") TRUE ("Discard?") _ _] -> w468
      tunnel: w463 -> [w482 w485 w498 w504 w510 w516 w528]
      tunnel: [_ _ w496 w509 _ w518 _] -> w466
      tunnel: [w482 w485 w497 w507 w510 w517 w528] -> w467
      tunnel: w451 -> [_ _ _ w502 _ w513 _]
      event Timeout {
        n173 = event-data() -> ()  [unwired: 1 in, 1 out]
        n174 = Wait (ms)(milliseconds to wait=u32 50) -> ()  [unwired: 1 out]
      }
      event Panel Resize {
        n175 = event-data() -> ("NewBnds"=w486:T13)  [unwired: 1 in]
        n176 = local read "Original Width"() -> (w487:u32)
        n177 = call "Front End Resize.vi"("Starting Font"=11.3, "Area to Font Division"=1300.0, "Original Text Box Width"=68, "NewBnds"=w486, "Original Panel Width"=w487) -> ("New Text Box Width"=w484:u64, "New Font Size"=w483:dbl)  [unwired: 5 in]
        n178 = flat-sequence {
          tunnel: w483 -> [w494]
          tunnel: w484 -> [w491]
          frame #0 {
            n179 = Multiply(x=w491, y=0.8) -> (x*y=w492:dbl)
            n180 = property on="User Name" class="Str"("Text.Width"=w492) -> ()  [unwired: 2 in, 2 out]
            n181 = property on="User Name" class="Str"("Text.FontSize"=w494) -> ()  [unwired: 2 in, 2 out]
          }
          frame #1 {
            n182 = property on="User Name" class="Str"("Text.SizeToText"=TRUE ("Text.Size to Text?")) -> ()  [unwired: 2 in, 2 out]
          }
        }
        n183 = property on="C" class="DigNum (strict)"("Label.FontSize"=w483) -> ()  [unwired: 2 in, 2 out]
        n184 = property on="g/min" class="DigNum (strict)"("Label.FontSize"=w483) -> ()  [unwired: 2 in, 2 out]
        n185 = property on="kg/m^3" class="DigNum (strict)"("Label.FontSize"=w483) -> ()  [unwired: 2 in, 2 out]
        n186 = property on="Total g" class="DigNum (strict)"("Label.FontSize"=w483) -> ()  [unwired: 2 in, 2 out]
        n187 = property on="C" class="DigNum (strict)"("NumText.FontSize"=w483) -> ()  [unwired: 2 in, 2 out]
        n188 = property on="g/min" class="DigNum (strict)"("NumText.FontSize"=w483) -> ()  [unwired: 2 in, 2 out]
        n189 = property on="kg/m^3" class="DigNum (strict)"("NumText.FontSize"=w483) -> ()  [unwired: 2 in, 2 out]
        n190 = property on="Total g" class="DigNum (strict)"("NumText.FontSize"=w483) -> ()  [unwired: 2 in, 2 out]
        n191 = property on="C" class="DigNum (strict)"("Text Width"=w484) -> ()  [unwired: 2 in, 2 out]
        n192 = property on="g/min" class="DigNum (strict)"("Text Width"=w484) -> ()  [unwired: 2 in, 2 out]
        n193 = property on="kg/m^3" class="DigNum (strict)"("Text Width"=w484) -> ()  [unwired: 2 in, 2 out]
        n194 = property on="Total g" class="DigNum (strict)"("Text Width"=w484) -> ()  [unwired: 2 in, 2 out]
      }
      event Panel Close? {
        w499 = TRUE  # Priority Message
        n195 = event-data() -> ()  [unwired: 1 in, 1 out]
        n196 = call-poly "Enqueue Message.vi"("Priority Message? (F)"=w499, "Message"="Confirm Quit", "Message Queue"=w498) -> ("error out"=w496:errorcluster, "dup Message Queue"=w497:refnum<queue>)  [unwired: 7 in]
        n197 = event-data("Discard?"=TRUE) -> ()  [unwired: 1 in, 1 out]
      }
      event "Exit": Value Change {
        w505 = TRUE  # Priority Message
        # "The UI Message Loop handles sending the Exit message to other loops."
        n198 = event-data() -> ()  [unwired: 1 in, 1 out]
        n199 = call "Generate Temporary Report.vi"("Line of Events"=string[] ["Exit Clicked"], "Module Name"=w502) -> ()  [unwired: 9 in, 1 out]
        n200 = call-poly "Enqueue Message.vi"("Priority Message? (F)"=w505, "Message"="Exit", "Message Queue"=w504) -> ("error out"=w509:errorcluster, "dup Message Queue"=w507:refnum<queue>)  [unwired: 7 in]
      }
      event User Event {
        # "The Message Handling Loop processed an \"Exit\" message, which fired this event to stop the Event Handling Loop."
        n201 = event-data() -> ()  [unwired: 1 in, 1 out]
        n202 = local write "Status"("Exit" ("Exit String")) -> ()
      }
      event "Settings Button": Mouse Down {
        n203 = event-data() -> ("PlatMods"=w515:T14)  [unwired: 1 in, 7 out]
        n204 = Unbundle By Name(w515) -> ("Ctrl"=w514:bool)
        n205 = case shown="False" w514 {
          tunnel: [w524 w525] -> w518
          tunnel: [w523 w526] -> w517
          tunnel: w516 -> [w522 w526]
          tunnel: w513 -> [w519 _]
          frame False {
            n206 = call "Generate Temporary Report.vi"("Line of Events"=string[] ["Settings Dialog Opened"], "Module Name"=w519) -> ()  [unwired: 9 in, 1 out]
            n207 = call-poly "Enqueue Message.vi"("Message"="Launch Settings Dialog", "Message Queue"=w522) -> ("error out"=w524:errorcluster, "dup Message Queue"=w523:refnum<queue>)  [unwired: 8 in]
          }
          frame True {
            n208 = property class="VI"("BDWin.Open"=TRUE ("Block Diagram Window:Open")) -> (error out=w525:errorcluster)  [unwired: 2 in, 1 out]
          }
        }
      }
      event Key Down {
        n209 = event-data() -> ("ScanCode"=→"ScanCode":i16)  [unwired: 1 in, 7 out]
      }
    }
    n210 = call "Error Handler - Event Handling Loop.vi"("error in (no error)"=w466, "Message Queue"=w467) -> ("dup error in"=w465:errorcluster, "dup Message Queue"=w453:refnum<queue>)  [unwired: 8 in]
  }
  n211 = call "Main Loop.vi"("error in (no error)"=w10, "Chart Notifier"=w16, "Message Queues"=w9) -> ("error out"=w17:errorcluster)  [unwired: 8 in]
  n212 = Release Queue(queue=w2) -> ()  [unwired: 2 in, 3 out]
  n213 = Close Reference(reference=w15) -> ()  [unwired: 1 in, 1 out]
  n214 = Unregister For Events(event registration refnum=w22, error in=w27) -> (error out=w23:errorcluster)
  n215 = Release Queue(queue=w4) -> ()  [unwired: 2 in, 3 out]
  n216 = Release Queue(queue=w3) -> ()  [unwired: 2 in, 3 out]
  n217 = Merge Errors(w23, w28, w10, w17) -> (w26:errorcluster)
  n218 = call "Destroy User Event - Stop.vi"("error in (no error)"=w26, "User Event - Stop"=w24) -> ("error out"=w6:errorcluster)  [unwired: 9 in]
  n219 = flat-sequence {
    tunnel: w6 -> [_]
    frame #0 {
      n220 = invoke class="VI" method="FP.Close"() -> ()  [unwired: 3 in, 3 out]
    }
  }
